vi "Data Write.vi"(7 "Retry Attempts (0)":i32 min=0, 8 "error in (no error)":errorcluster, 10 "Command":string, 11 "VISA Refnum in":refnum<visa-resource-name>) -> (0 "error out":errorcluster, 3 "VISA Refnum out":refnum<visa-resource-name>)   [LabVIEW 2020, in "ChromTech Series I Drivers.lvlib"]
doc: "Performs a VISA Write to the given VISA port with the given command. The write action will be retried upon failure up to N times, where N is the Retry Attempts given, where N >= 0. Values less than zero will be treated as zero. The first wait time is 1 second, which doubles in subsequent retry wait times, similar to TCP communications prior to any segments being received.\n\nFor example, attempt 1 (0 retries) = 1 second wait; attempt 2 (1 retry) = 2 second wait; attempt 3 (2 retries) = 4 second wait. The number of seconds waited on a given retry attempt can be represented with the formula 2^n, where n is the number of retries attempted."
uses:
  <instrlib>/RxnRover/ChromtechSeriesIDriver/ChromTech Series I Drivers.lvlib
  <vilib>/Utility/sysdir.llb/System Directory Type.ctl
panel:
  out "Retries":i32
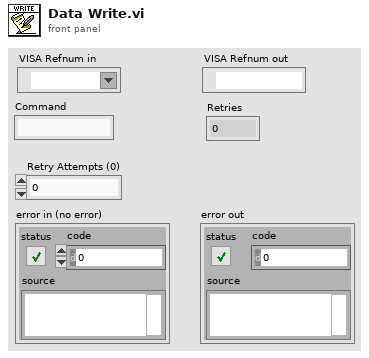
[diagram p1: front panel]
types:
  T1 = typedef "System Directory Type.ctl" = i32
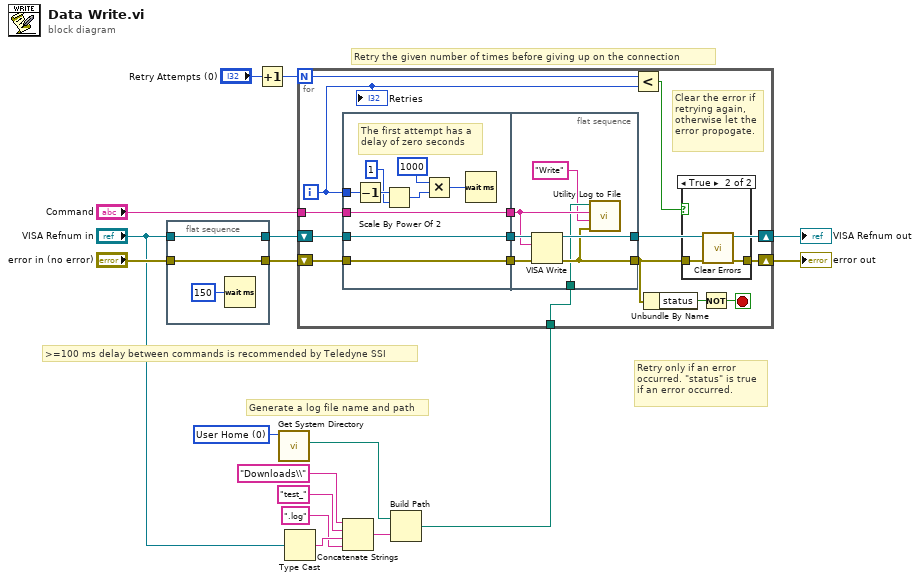
[diagram p0: block diagram]
diagram:
  w8 = T1 0 items=["User Home"=0, "User Desktop"=1, "User Documents"=2, "User Application Data"=3, "User Preferences"=4, "User Temporary"=5, "Public Documents"=6, "Public Application Data"=7, "Public Preferences"=8, "Public Cache"=13, "System Core Libraries"=9, "System Installed Libraries"=10, "Application Files"=11, "Boot Volume Root"=12] ("system directory type")
  # "Retry only if an error\noccurred. \"status\" is true\nif an error occurred."
  # "Retry the given number of times before giving up on the connection"
  # "Generate a log file name and path"
  # ">=100 ms delay between commands is recommended by Teledyne SSI"
  n1 = flat-sequence {
    tunnel: "error in (no error)" -> [w20]
    tunnel: "VISA Refnum in" -> [w19]
    tunnel: [w19] -> w15
    tunnel: [w20] -> w14
    frame #0 {
      n2 = Wait (ms)(milliseconds to wait=u32 150) -> ()  [unwired: 1 out]
    }
  }
  n3 = Increment(x="Retry Attempts (0)") -> (x+1=w1:i32)
  n4 = call <vilib>:"Get System Directory.vi"("system directory type"=w8) -> ("system directory"=w4:path)  [unwired: 10 in]
  n5 = Type Cast(x="VISA Refnum in") -> (*(type *) &x=w10:string)  [unwired: 1 in]
  n6 = Concatenate Strings("Downloads\\", "test_", w10, ".log") -> (w5:string)
  n7 = Build Path(base path=w4, name or relative path=w5) -> (appended path=w3:path)
  n8 = for {
    N: w1 -> [w22]
    tunnel: "Command" -> [w32]
    tunnel: w3 -> [w28]
    shift-right: [w35] -> w17
    shift-left: w15 -> [w34]
    shift-right: [w24] -> w12
    shift-left: w14 -> [w33]
    i -> [w21]
    stop <- w25 stop-if-true
    # "Clear the error if\nretrying again,\notherwise let the\nerror propogate."
    n9 = flat-sequence {
      tunnel: w32 -> [w45]
      tunnel: w33 -> [w46]
      tunnel: w34 -> [w47]
      tunnel: [w47] -> w31
      tunnel: [w46] -> w30
      tunnel: [w45] -> w29
      tunnel: w21 -> [w44]
      tunnel: [w54] -> w35
      tunnel: [w51] -> w27
      tunnel: w28 -> [w49]
      tunnel: w31 -> [w53]
      tunnel: w30 -> [w52]
      tunnel: w29 -> [w50]
      frame #0 {
        # "The first attempt has a \ndelay of zero seconds"
        n10 = Decrement(x=w44) -> (x-1=w40:i32)
        n11 = Scale By Power Of 2(n=w40, x=1) -> (x*2^n=w43:i32)
        n12 = Multiply(x=1000, y=w43) -> (x*y=w41:i32)
        n13 = Wait (ms)(milliseconds to wait=w41) -> ()  [unwired: 1 out]
      }
      frame #1 {
        n14 = VISA Write(VISA resource name=w53, write buffer=w50, error in (no error)=w52) -> (VISA resource name out=w54:refnum<visa-resource-name>, error out=w51:errorcluster)  [unwired: 1 out]
        n15 = call <instrlib>:"Utility Log to File.vi"("error in (no error)"=w51, "Additional Notes"="Write", "Command"=w50, "Log File Path"=w49) -> ()  [unwired: 7 in, 1 out]
      }
    }
    n16 = Less?(x=w22, y=w21) -> (x < y?=w23:bool)
    n17 = Unbundle By Name(w27) -> ("status"=w26:bool)
    n18 = case shown="True" w23 {
      tunnel: w27 -> [w36 w38]
      tunnel: [w36 w37] -> w24
      frame False {
      }
      frame True {
        n19 = call <vilib>:"Clear Errors.vi"("error in (no error)"=w38) -> ("error out"=w37:errorcluster)  [unwired: 5 in, 1 out]
      }
    }
    n20 = Not(x=w26) -> (.not. x?=w25:bool)
    "Retries" <- w21
  }
  "VISA Refnum out" <- w17
  "error out" <- w12
